vi "PathPlanner_TrajectoryWaypoint_New.vi"(6 "IsReversed":bool, 7 "AnchorPoint":T1 {"Y" format="%14.3f"; "X" format="%14.3f"}, 8 "HolonomicRotation":T3={"VALUE"=0.0, "COS"=1.0, "SIN"=0.0} {"SIN" format="%13.4f"; "COS" format="%13.4f"; "VALUE" format="%13.4f"}, 9 "VelOverride":dbl, 10 "NextControl":T1 {"Y" format="%14.3f"; "X" format="%14.3f"}, 11 "PrevControl":T1 {"Y" format="%14.3f"; "X" format="%14.3f"}) -> (3 "PathPlannerWaypoint":T2={"AnchorPoint"={"X"=0.0, "Y"=0.0}, "PrevControl"={"X"=0.0, "Y"=0.0}, "NextControl"={"X"=0.0, "Y"=0.0}, "HolonomicRotation"={"VALUE"=0.0, "COS"=1.0, "SIN"=0.0}, "VelOverride"=0.0, "isReversal"=FALSE} {"HolonomicRotation"."SIN" format="%13.4f"; "HolonomicRotation"."COS" format="%13.4f"; "HolonomicRotation"."VALUE" format="%13.4f"; "NextControl"."Y" format="%14.3f"; "NextControl"."X" format="%14.3f"; "PrevControl"."Y" format="%14.3f"; "PrevControl"."X" format="%14.3f"; "AnchorPoint"."Y" format="%14.3f"; "AnchorPoint"."X" format="%14.3f"})   [LabVIEW 2019, in "PathPlanner24.lvlib"]
uses:
  PathPlanner24.lvlib
  <vilib>/Rock Robotics/WPI/ThirdParty/JAS_Junk/TrajLib/TypeDef/TRANSLATION2D.ctl
  <vilib>/Rock Robotics/WPI/ThirdParty/JAS_Junk/TrajLib/TypeDef/ROTATION2D.ctl
  TypeDef/PathPlannerWaypoint.ctl
  <vilib>/Rock Robotics/WPI/ThirdParty/JAS_Junk/TrajLib/Trajectory_Library.lvlib
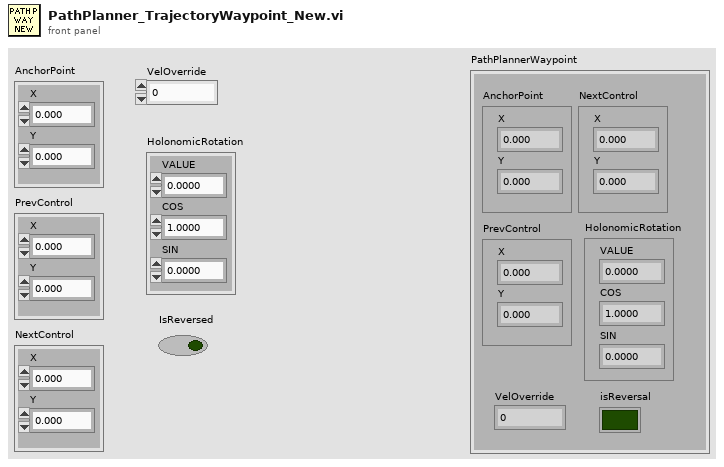
[diagram p1: front panel]
types:
  T1 = typedef "Trajectory_Library.lvlib/TRANSLATION2D.ctl" = cluster{"X":dbl, "Y":dbl}
  T2 = typedef "PathPlanner24.lvlib/PathPlannerWaypoint.ctl" = cluster{"AnchorPoint":T1, "PrevControl":T1, "NextControl":T1, "HolonomicRotation":T3, "VelOverride":dbl, "isReversal":bool}
  T3 = typedef "Trajectory_Library.lvlib/ROTATION2D.ctl" = cluster{"VALUE":dbl, "COS":dbl, "SIN":dbl}
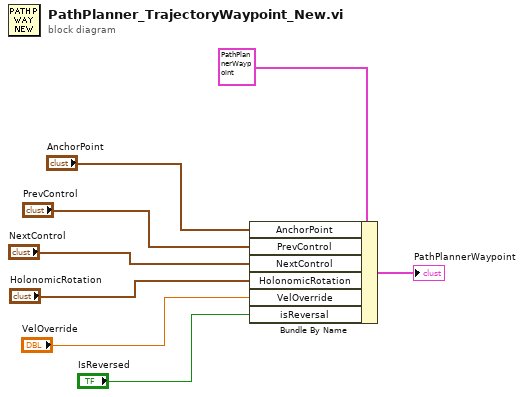
[diagram p0: block diagram]
diagram:
  n1 = Bundle By Name(cluster=T2 {"AnchorPoint"={"X"=0.0, "Y"=0.0}, "PrevControl"={"X"=0.0, "Y"=0.0}, "NextControl"={"X"=0.0, "Y"=0.0}, "HolonomicRotation"={"VALUE"=0.0, "COS"=1.0, "SIN"=0.0}, "VelOverride"=0.0, "isReversal"=FALSE} ("PathPlannerWaypoint"), "AnchorPoint"="AnchorPoint", "PrevControl"="PrevControl", "NextControl"="NextControl", "HolonomicRotation"="HolonomicRotation", "VelOverride"="VelOverride", "isReversal"="IsReversed") -> (→"PathPlannerWaypoint":T2)
